vi "3.7-UDP Where Server.vi"() -> ()   [LabVIEW 2010]
doc: "Creates a named service and listens on the first available port. Whenever a client connects to the service, it responds with a message containing joystick data. The VI can be stopped using the STOP button."
uses:
  3.2-Where/_typedefs/3.2-Where Sensor Typedef.ctl
  4-High Neurons/Current GPS Data.ctl
  3.2-Where/_typedefs/3.2.1-VectorNav Data.ctl
  3.0-Global.vi
panel:
  out "Where Data Am I":T1 {"4.2.2-GPS Data"."Longitude (dd.mmmmmm)" format="%#.6g"; "4.2.2-GPS Data"."Lattitude (dd.mmmmmm)" format="%#.6g"}
  out "data out":string
  out "error out":errorcluster
  in  "error in":errorcluster
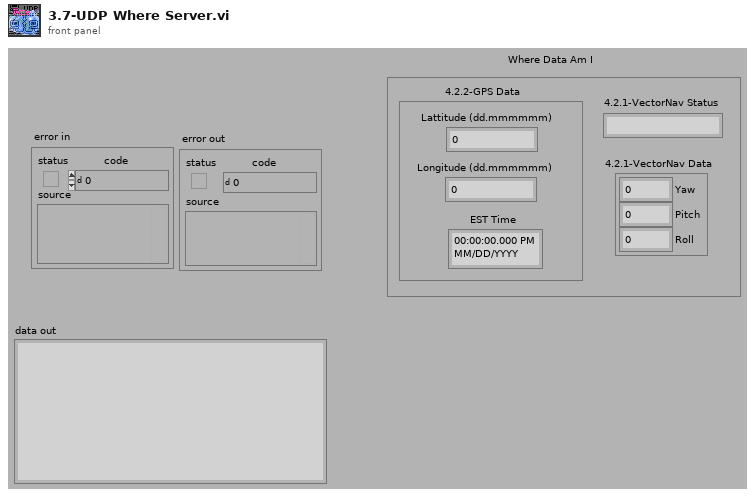
[diagram p1: front panel]
types:
  T1 = typedef "3.2-Where Sensor Typedef.ctl" = cluster{"4.2.2-GPS Data":T2, "4.2.1-VectorNav Data":T3, "4.2.1-VectorNav Status":string}
  T2 = typedef "Current GPS Data.ctl" = cluster{"Lattitude (dd.mmmmmm)":dbl, "Longitude (dd.mmmmmm)":dbl, "EST Time":timestamp}
  T3 = typedef "3.2.1-VectorNav Data.ctl" = cluster{"Yaw":dbl, "Pitch":dbl, "Roll":dbl}
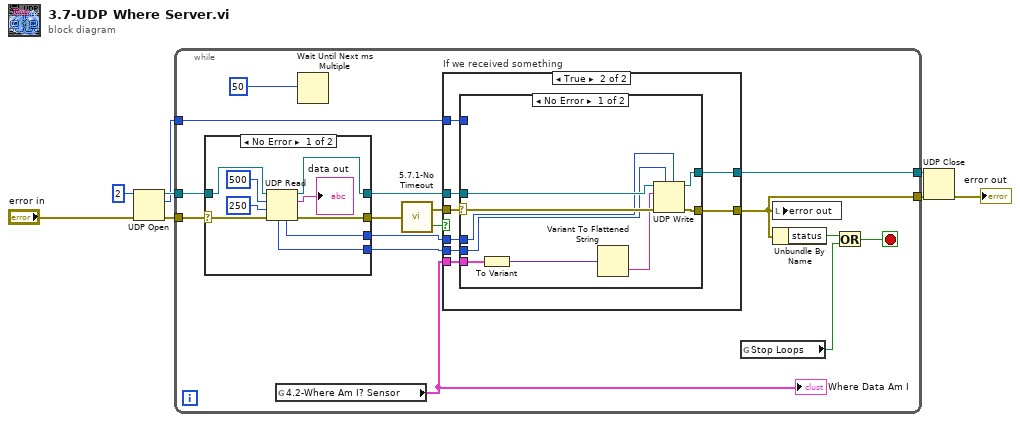
[diagram p0: block diagram]
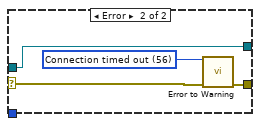
[diagram p3: hidden frame]
diagram:
  n1 = UDP Open(8:"error in", 11:u16 2 ("port")) -> (port=w7:refnum<k16>, 0:w6:errorcluster, 2:w2:u16)  [unwired: 3 in]
  n2 = while {
    tunnel: [w13] -> w4
    tunnel: w7 -> [w24]
    tunnel: w6 -> [w21]
    tunnel: [w22] -> w5
    tunnel: w2 -> [w18]
    stop <- w16 stop-if-true
    n3 = case shown="No Error" w21 {
      selector: w21 -> [w54 w57]
      tunnel: w24 -> [w56 w58]
      tunnel: [w53 w58] -> w23
      tunnel: [w52 w57] -> w12
      tunnel: [w50 _] -> w19
      tunnel: [w51 _] -> w20
      frame No Error {
        n4 = UDP Read(connection ID=w56, max size (548)=500, timeout ms (25000)=250, 8:w54) -> (data out=→"data out":string, error out=w52:errorcluster, 3:w53:refnum<k16>, 4:w50:u16, 6:w51:u32)
      }
      frame Error {
      }
    }
    n5 = global read "3.0-Global.vi" "4.2-Where Am I? Sensor"() -> (w10:T1)
    "Where Data Am I" <- w10
    n6 = Wait Until Next ms Multiple(millisecond multiple=u32 50 ("milliseconds to wait")) -> ()  [unwired: 1 out]
    n7 = call "5.7.1-No Timeout.vi"("error in (no error)"=w12) -> ("No Timeout"=w14:bool, "error out"=w15:errorcluster)
    n8 = case "If we received something" shown="True" w14 {
      tunnel: w23 -> [w25 w34]
      tunnel: [w25 w33] -> w22
      tunnel: w20 -> [_ w32]
      tunnel: w19 -> [_ w31]
      tunnel: w18 -> [_ w30]
      tunnel: [w26 w29] -> w13
      tunnel: w15 -> [w26 w28]
      tunnel: w10 -> [_ w27]
      frame False {
      }
      frame True {
        n9 = case shown="No Error" w28 {
          selector: w28 -> [w43 w45]
          tunnel: w34 -> [w40 w47]
          tunnel: [w42 w44] -> w29
          tunnel: [w41 w47] -> w33
          tunnel: w32 -> [w38 _]
          tunnel: w31 -> [w39 _]
          tunnel: w30 -> [_ _]
          tunnel: w27 -> [w35 _]
          frame No Error {
            n10 = To Variant(anything=w35) -> (Variant=w37:variant)
            n11 = Variant To Flattened String(Variant=w37) -> (data string=w36:string)  [unwired: 1 out]
            n12 = UDP Write(address=w38, port or service name=w39, connection ID=w40, data in=w36, 8:w43) -> (error out=w42:errorcluster, 3:w41:refnum<k16>)  [unwired: 1 in]
          }
          frame Error {
            w46 = 56 items=["No Error", "Argument Error", "Memory Full", "Out of Zone", "End of File", "File Already Open", "Generic File IO Error", "File Not Found", "File Permission Error", "Disk Full", "Duplicate Path", "Too Many Files Open", "Not Enabled", "Resource File Not Found", "Cannot Add Resource", "Resource Not Found", "Image Not Found", "Image Memory Error", "Pen Does Not Exist", "Config Bad Type", "Config Token Not Found", "Config Parse Error", "Config Memory Error", "Bad External Code Format", "Bad External Code Offset", "External Code Not Present", "Null Window", "Destroy Window Mixup", "Null Menu", "Print Aborted", "Bad Print Record", "Print Driver Error", "Windows Error During Print", "Memory Error During Print", "Print Dialog Error", "Generic Print Error", "Invalid Device Refnum", "Device Not Found", "Device Parameter Error", "Device Unit Error", "Can't Open Device", "Device Call Aborted", "Generic Error", "Cancelled By User", "Object ID Too Low", "Object ID Too High", "Object Not In Heap", "Unknown Heap", "Bad DefProc ID", "DefProc Not In Table", "Message Out Of Range", "Null Method", "Unknown Message", "Manager Call Not Supported", "Bad address", "Connection In progress", "Connection timed out", "Connection is already in progress", "Network attribute not supported", "Network error", "Address in use", "System out of memory", "Connection aborted", "Connection refused", "Connection is not connected", "Connection is already connected", "Connection closed", "Initialize error (interapplication manager)", "Bad occurrence", "Wait on unbound occurrence handler", "Occurrence queue overflow", "Bad path", "Semaphore not signaled", "Unrecognized type (interapplication manager)"] ("1st Error to Convert")
            n13 = call <vilib>:"Error to Warning.vi"("1st Error to Convert"=w46, "error in"=w45) -> ("warning out"=w44:errorcluster)  [unwired: 13 in]
          }
        }
      }
    }
    n14 = global read "3.0-Global.vi" "Stop Loops"() -> (w11:bool)
    n15 = local write "error out"(w13) -> ()
    n16 = Unbundle By Name(w13) -> ("status"=w17:bool)
    n17 = Or(x=w17, y=w11) -> (x .or. y?=w16:bool)
  }
  n18 = UDP Close(connection ID=w5, 8:w4) -> (error out=→"error out":errorcluster)  [unwired: 1 out]
